vi "IECal-Restore Defaults.vi"(11 "error in (no error)":errorcluster) -> (8 "Params":T1={"Speaker"="", "Stimulus"={"Type"="", "Freq step (Hz)"=50000.0, "Sampling rate (Hz)"=50.0, "Attenuation (dB)"=0.0}, "Averages"=0, "Left gain"=0.0, "Right gain"=0.0, "plot max"=FALSE, "Max Vmic"=0.0}, 15 "error out":errorcluster)   [LabVIEW 2020]
uses:
  Typedefs/IECal-Parameters.ctl
  Common VIs/Typedefs/CAL-Stimulus.ctl
  bb9e3314-2d63-47a2-bbf4-cdf68ae0e619.vi
  epl-vi-lib/Utility VIs/File IO VIs/Read Write Anything/Read Anything.vi
panel:
  in  "Defaults":T1={"Speaker"="Right primary", "Stimulus"={"Type"="Chirp", "Freq step (Hz)"=50000.0, "Sampling rate (Hz)"=50.0, "Attenuation (dB)"=30.0}, "Averages"=250, "Left gain"=40.0, "Right gain"=40.0, "plot max"=FALSE, "Max Vmic"=6.0}
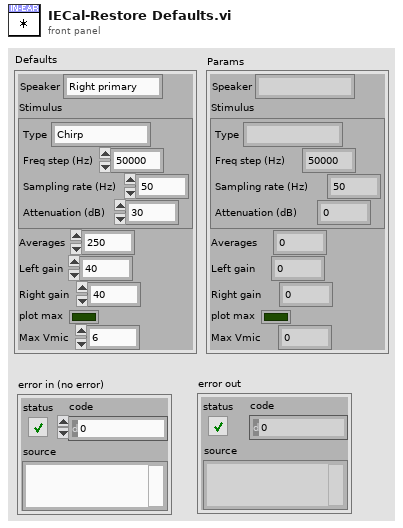
[diagram p1: front panel]
types:
  T1 = typedef "IECal-Parameters.ctl" = cluster{"Speaker":string, "Stimulus":T2, "Averages":i32, "Left gain":dbl, "Right gain":dbl, "plot max":bool, "Max Vmic":dbl}
  T2 = typedef "CAL-Stimulus.ctl" = cluster{"Type":string, "Freq step (Hz)":dbl, "Sampling rate (Hz)":dbl, "Attenuation (dB)":dbl}
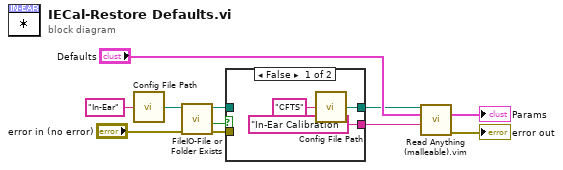
[diagram p0: block diagram]
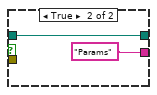
[diagram p2: hidden frame]
diagram:
  n1 = call "Config File Path.vi"("AppName"="In-Ear") -> ("Default config file name"=w10:path)
  n2 = call "FileIO-File or Folder Exists.vi"("error in (no error)"="error in (no error)", "path"=w10) -> ("error out"=w4:errorcluster, "Exists?"=w3:bool, "dup path"=w5:path)  [unwired: 6 in, 1 out]
  n3 = case shown="False" w3 {
    tunnel: w5 -> [_ w15]
    tunnel: w4 -> [_ _]
    tunnel: ["In-Ear Calibration" ("Section Name (Name of \"Anything\")") "Params" ("Section Name (Name of \"Anything\")")] -> w2
    tunnel: [w13 w15] -> w1
    frame False {
      n4 = call "Config File Path.vi"("AppName"="CFTS") -> ("Default config file name"=w13:path)
    }
    frame True {
    }
  }
  n5 = call "Read Anything (malleable).vim"("Config file path"=w1, "Options in"="Defaults", "Section"=w2) -> ("Options out"=→"Params":T1, "error out"=→"error out":errorcluster)  [unwired: 10 in, 1 out]
